vi "FdxCmdRxVLGetActivityCvi.vi"(8 "error in":errorcluster, 9 "Input Cluster":T2 {"Mode" items=["FDX_RX_VL_ACT_ALL", "FDX_RX_VL_ACT_VL", "FDX_RX_VL_ACT_CNT"]}, 11 "InstrumentHandle_port":u32) -> (0 "error out":errorcluster, 1 "VLActivityOut":T1, 3 "InstrumentHandle_port":u32)   [LabVIEW 2020, in "AIM664LV.lvlib"]
doc: "This function is used to obtain the activity status for all active or a specific Virtual Link(s). The memory which is needed for this list has to be provided by the application."
uses:
  AIM664LV.lvlib
  AFDX_LibraryAdmin/FdxGlobalDllPath.vi
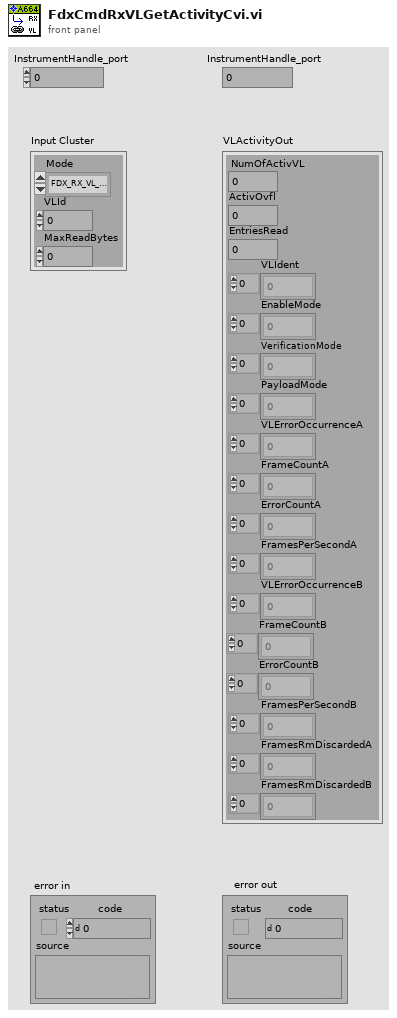
[diagram p1: front panel]
types:
  T1 = cluster{"NumOfActivVL":u32, "ActivOvfl":u32, "EntriesRead":u32, "VLIdent":u32[], "EnableMode":u32[], "VerificationMode":u32[], "PayloadMode":u32[], "VLErrorOccurrenceA":u32[], "FrameCountA":u32[], "ErrorCountA":u32[], "FramesPerSecondA":u32[], "VLErrorOccurrenceB":u32[], "FrameCountB":u32[], "ErrorCountB":u32[], "FramesPerSecondB":u32[], "FramesRmDiscardedA":u32[], "FramesRmDiscardedB":u32[]}
  T2 = cluster{"Mode":u32, "VLId":u32, "MaxReadBytes":u32}
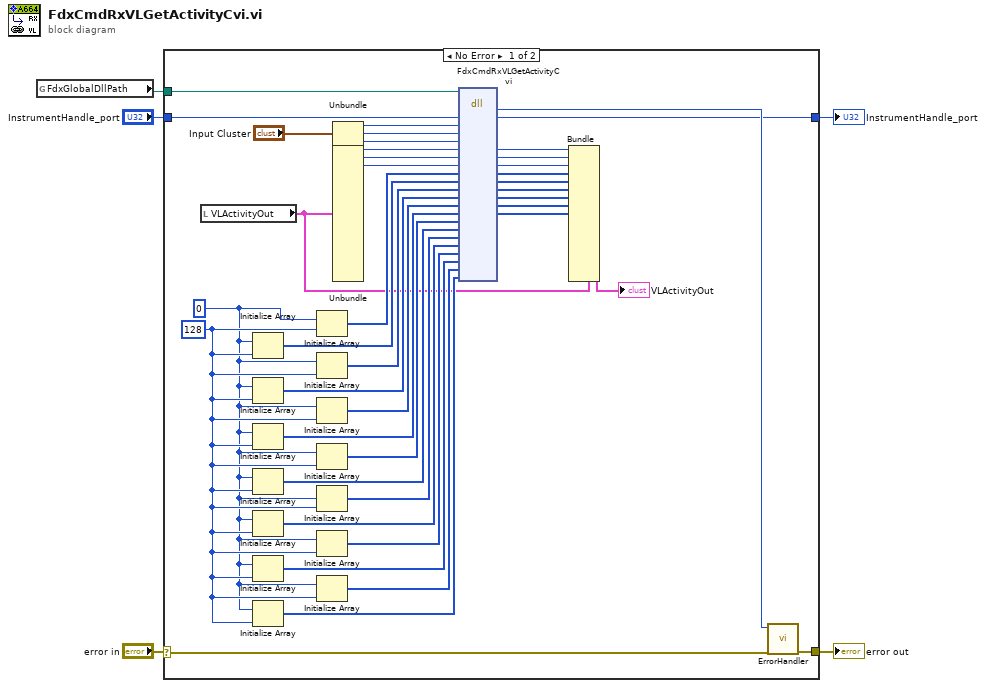
[diagram p0: block diagram]
diagram:
  n1 = global read "FdxGlobalDllPath.vi" "FdxGlobalDllPath"() -> (w3:path)
  n2 = case shown="No Error" "error in" {
    selector: "error in" -> [w44 w47]
    tunnel: [w45 w47] -> w5
    tunnel: w3 -> [w8 _]
    tunnel: "InstrumentHandle_port" -> [w7 w46]
    tunnel: [w6 w46] -> w1
    frame No Error {
      w25 = 128 ("dimension size")
      w24 = u32 0 ("element")
      n3 = local read "VLActivityOut"() -> (w9:T1)
      n4 = Initialize Array(w24, w25) -> (w27:u32[])
      n5 = Initialize Array(w24, w25) -> (w23:u32[])
      n6 = Initialize Array(w24, w25) -> (w21:u32[])
      n7 = Initialize Array(w24, w25) -> (w19:u32[])
      n8 = Initialize Array(w24, w25) -> (w17:u32[])
      n9 = Initialize Array(w24, w25) -> (w15:u32[])
      n10 = Initialize Array(w24, w25) -> (w13:u32[])
      n11 = Initialize Array(w24, w25) -> (w28:u32[])
      n12 = Initialize Array(w24, w25) -> (w26:u32[])
      n13 = Initialize Array(w24, w25) -> (w22:u32[])
      n14 = Initialize Array(w24, w25) -> (w20:u32[])
      n15 = Initialize Array(w24, w25) -> (w18:u32[])
      n16 = Initialize Array(w24, w25) -> (w16:u32[])
      n17 = Initialize Array(w24, w25) -> (w14:u32[])
      n18 = Unbundle("Input Cluster") -> ("Mode"=w41:u32, "VLId"=w40:u32, "MaxReadBytes"=w39:u32)
      n19 = Unbundle(w9) -> ("NumOfActivVL"=w12:u32, "ActivOvfl"=w11:u32, "EntriesRead"=w10:u32)  [unwired: 14 out]
      n20 = dll-call lib="aim_fdx.19.dll" fn="FdxCmdRxVLGetActivityCvi"(path in=w8, "InstrumentHandle"=w7, "Mode"=w41, "VLId"=w40, "MaxReadBytes"=w39, "NumOfActivVL"=w12, "ActivOvfl"=w11, "EntriesRead"=w10, "VLIdent"=w28, "EnableMode"=w27, "VerificationMode"=w26, "PayloadMode"=w23, "VLErrorOccurrenceA"=w22, "FrameCountA"=w21, "ErrorCountA"=w20, "FramesPerSecondA"=w19, "VLErrorOccurrenceB"=w18, "FrameCountB"=w17, "ErrorCountB"=w16, "FramesPerSecondB"=w15, "FramesRmDiscardedA"=w14, "FramesRmDiscardedB"=w13) -> ("status"=w43:i32, "InstrumentHandle"=w6:u32, "NumOfActivVL"=w38:u32, "ActivOvfl"=w37:u32, "EntriesRead"=w36:u32, "VLIdent"=w31:u32[], "EnableMode"=w29:u32[], "VerificationMode"=w32:u32[], "PayloadMode"=w33:u32[], "VLErrorOccurrenceA"=w34:u32[], "FrameCountA"=w35:u32[])  [unwired: 5 in, 10 out]
      n21 = Bundle(cluster=w9, "NumOfActivVL"=w38, "ActivOvfl"=w37, "EntriesRead"=w36, "VLIdent"=w31, "EnableMode"=w29, "VerificationMode"=w32, "PayloadMode"=w33, "VLErrorOccurrenceA"=w34, "FrameCountA"=w35) -> (→"VLActivityOut":T1)  [unwired: 8 out]
      n22 = call "ErrorHandler.vi"("error in"=w44, "AIM Error"=w43) -> ("error out"=w45:errorcluster)  [unwired: 9 in]
    }
    frame Error {
    }
  }
  "error out" <- w5
  "InstrumentHandle_port" <- w1
